vi "Meas Result Release Access.vi"(7 "timout [s] (30s)":dbl=30.0 format="%#_13g", 8 "error in":errorcluster, 9 "Release only (True)":bool=TRUE, 10 "results data in":T1, 11 "results ref":refnum<vi>) -> (0 "error out":errorcluster)   [LabVIEW 2020]
doc: "Call this to release exclusive access to the result. Use the flag 'release only' to not store the result data."
uses:
  Meas Results.ctl
  bridge/Bridge Frequency Readings Data.ctl
  drivers/TWM client/Meas Proc QWTB Spectrum Data.ctl
  drivers/TWM client/TWM Phase Info.ctl
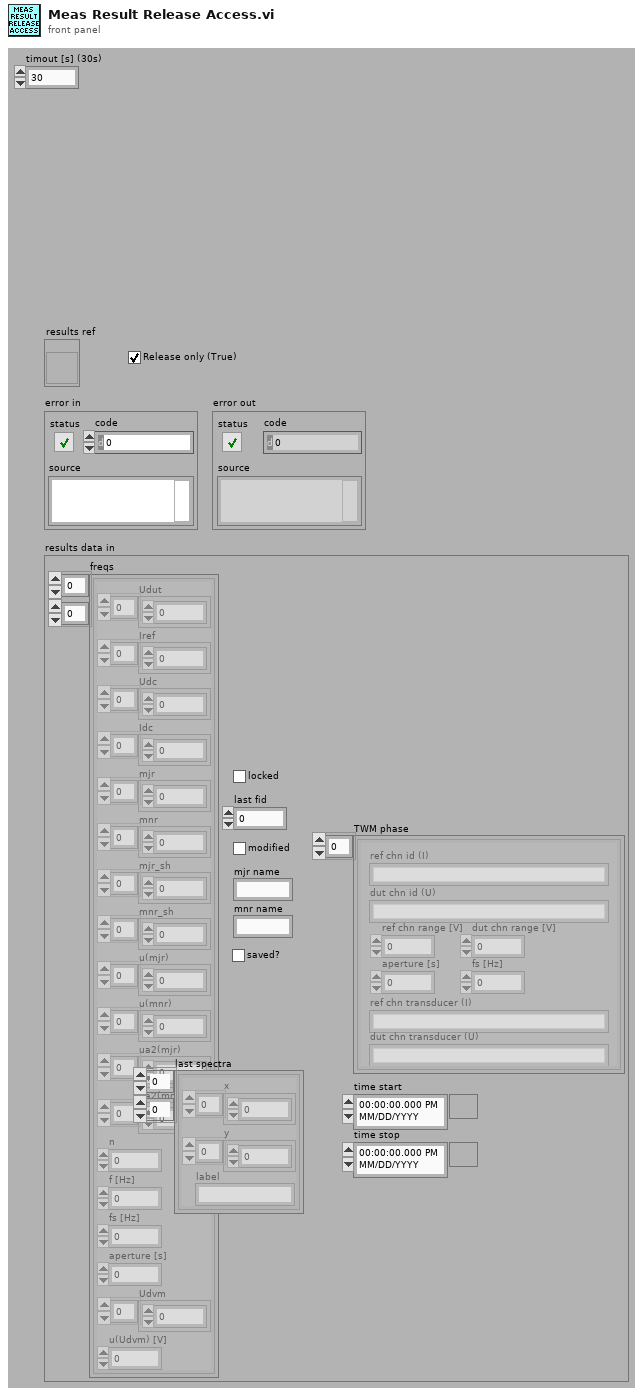
[diagram p1: front panel]
types:
  T1 = typedef "Meas Results.ctl" = cluster{"freqs":T2[][], "locked":bool, "last fid":i32, "modified":bool, "mjr name":string, "mnr name":string, "last spectra":T3[][], "saved?":bool, "TWM phase":T4[], "time start":timestamp, "time stop":timestamp}
  T2 = typedef "Bridge Frequency Readings Data.ctl" = cluster{"Udut":dbl[], "Iref":dbl[], "Udc":dbl[], "Idc":dbl[], "mjr":dbl[], "mnr":dbl[], "mjr_sh":dbl[], "mnr_sh":dbl[], "u(mjr)":dbl[], "u(mnr)":dbl[], "ua2(mjr)":dbl[], "ua2(mnr)":dbl[], "n":i32, "f [Hz]":dbl, "fs [Hz]":dbl, "aperture [s]":dbl, "Udvm":dbl[], "u(Udvm) [V]":dbl}
  T3 = typedef "Meas Proc QWTB Spectrum Data.ctl" = cluster{"x":sgl[], "y":sgl[], "label":string}
  T4 = typedef "TWM Phase Info.ctl" = cluster{"ref chn id (I)":string, "dut chn id (U)":string, "ref chn range [V]":dbl, "dut chn range [V]":dbl, "aperture [s]":dbl, "fs [Hz]":dbl, "ref chn transducer (I)":string, "dut chn transducer (U)":string}
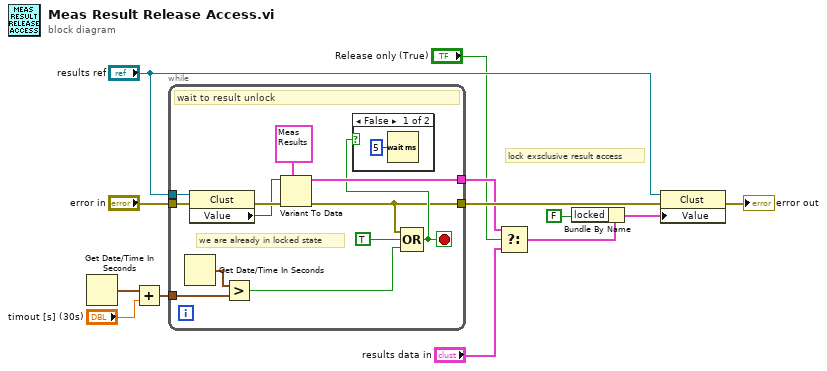
[diagram p0: block diagram]
diagram:
  # "lock exsclusive result access"
  n1 = Get Date/Time In Seconds() -> (seconds since 1Jan1904=w11:timestamp)
  n2 = Add(x=w11, y="timout [s] (30s)") -> (x+y=w9:timestamp)
  n3 = while {
    tunnel: "results ref" -> [w25]
    tunnel: "error in" -> [w24]
    tunnel: [w15] -> w8
    tunnel: [w20] -> w4
    tunnel: w9 -> [w18]
    stop <- w16 stop-if-true
    # "we are already in locked state"
    # "wait to result unlock"
    n4 = Get Date/Time In Seconds() -> (seconds since 1Jan1904=w19:timestamp)
    n5 = property class="Clust"(reference=w25, error in=w24) -> (error out=w23:errorcluster, "Value"=w22:variant)  [unwired: 1 out]
    n6 = Greater?(x=w19, y=w18) -> (0:w17:bool)
    n7 = Variant To Data(error in=w23, type=T1 {"freqs"=[], "locked"=FALSE, "last fid"=0, "modified"=FALSE, "mjr name"="", "mnr name"="", "last spectra"=[], "saved?"=FALSE, "TWM phase"=[], "time start"=timestamp(0 s since 1904-01-01), "time stop"=timestamp(0 s since 1904-01-01)} ("Cluster"), Variant=w22) -> (data=w20:T1, error out=w15:errorcluster)
    n8 = Compound Arithmetic op=OR(w15, TRUE, w17) -> (w16:bool)
    n9 = case shown="False" w16 {
      frame False {
        n10 = Wait (ms)(milliseconds to wait=u32 5) -> ()  [unwired: 1 out]
      }
      frame True {
      }
    }
  }
  n11 = Select(t=w4, s="Release only (True)", f="results data in") -> (s? t:f=w1:T1)
  n12 = Bundle By Name(cluster=w1, "locked"=FALSE) -> (w5:T1)
  n13 = property class="Clust"(reference="results ref", error in=w8, "Value"=w5) -> (error out=→"error out":errorcluster)  [unwired: 1 out]
